vi "SJ_Signal_Smooth.vi"(2 "Sampling Frequency":dbl=-999.0 format="%.2f", 3 "Jet Frequency":dbl, 4 "Signal":dbl[](array[numeric]) format="%0.2f") -> (1 "Smoothed Signal":dbl[](array[numeric]))   [LabVIEW 2011]
uses:
  <vilib>/Analysis/3filter.llb/Filter Passband Type.ctl
  <vilib>/Analysis/3filter.llb/Filter Structure Type.ctl
  <vilib>/Analysis/baseanly.llb/Scale 1D.vi
  <vilib>/Analysis/3filter.llb/Zero Phase Filter (obs, DBL).vi
  <vilib>/Analysis/NI_AALBase.lvlib
  <vilib>/Analysis/NI_AALPro.lvlib
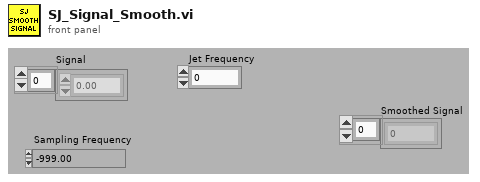
[diagram p1: front panel]
types:
  T1 = typedef "NI_AALBase.lvlib/Filter Structure Type.ctl" = u16
  T2 = typedef "NI_AALBase.lvlib/Filter Passband Type.ctl" = enum32{"Lowpass", "Highpass", "Bandpass", "Bandstop"}
  T3 = cluster{"filter structure":enum32{"IIR 2nd Order", "IIR 4th Order"}, "Reverse Coefficients":dbl[], "Forward Coefficients":dbl[]}
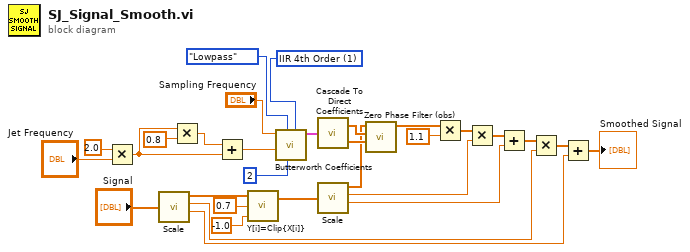
[diagram p0: block diagram]
diagram:
  w25 = T1 1 items=["IIR 2nd Order"=0, "IIR 4th Order"=1, "Auto Select"=10] ("filter structure option")
  n1 = Multiply(x=2.0, y="Jet Frequency") -> (x*y=w28:dbl)
  n2 = call-poly <vilib>:"Scale.vi"("X"="Signal") -> ("Y=(X-offset)/scale"=w18:dbl[], "scale"=w10:dbl, "offset"=w9:dbl)  [unwired: 1 out]
  n3 = Multiply(x=w28, y=0.8) -> (x*y=w27:dbl)
  n4 = Add(x=w27, y=w28) -> (x+y=w22:dbl)
  n5 = call <vilib>:"Y[i]=Clip{X[i]}.vi"("lower limit"=-1.0, "upper limit"=0.7, "Input Array"=w18) -> ("Clipped Array"=w16:dbl[])  [unwired: 1 out]
  n6 = call <vilib>:"Butterworth Coefficients.vi"("filter structure option"=w25, "order"=2, "filter type"=Filter_Passband_Type."Lowpass", "low cutoff freq: fl"=w22, "sampling freq: fs"="Sampling Frequency") -> ("IIR Filter Cluster"=w24:T3)  [unwired: 5 in, 1 out]
  n7 = call <vilib>:"Cascade To Direct Coefficients.vi"("IIR Filter Cluster"=w24) -> ("Reverse Coefficients"=w23:dbl[], "Forward Coefficients"=w20:dbl[])
  n8 = call-poly <vilib>:"Scale.vi"("X"=w16) -> ("Y=(X-offset)/scale"=w15:dbl[], "scale"=w14:dbl, "offset"=w13:dbl)  [unwired: 1 out]
  n9 = call-poly <vilib>:"Zero Phase Filter (obs).vi"("Forward Coefficients"=w20, "Reverse Coefficients"=w23, "X"=w15) -> ("Filtered X"=w8:dbl[])  [unwired: 7 in, 1 out]
  n10 = Multiply(x=w8, y=1.1) -> (x*y=w7:dbl[])
  n11 = Multiply(x=w7, y=w14) -> (x*y=w17:dbl[])
  n12 = Add(x=w17, y=w13) -> (x+y=w11:dbl[])
  n13 = Multiply(x=w11, y=w10) -> (x*y=w12:dbl[])
  n14 = Add(x=w12, y=w9) -> (x+y=→"Smoothed Signal":dbl[])
